vi "REQ-REP.vi"() -> ()   [LabVIEW 2018]
uses:
  RxTx/CM_RxTx.lvclass
  socket REQ/socket REQ.lvclass
  C:/Users/Denis/Desktop/communication-manager/communication-manager/Socket/Socket.lvclass
  socket REP/socket REP.lvclass
  Socket/Socket.lvclass
  <vilib>/addons/zeromq/zmq_context.lvclass
panel:
  in  "socket REP.lvclass":refnum<class "socket REP.lvclass">
  in  "socket REQ.lvclass":refnum<class "socket REQ.lvclass">
  out "error out 3":errorcluster
  in  "Queue RX 2":refnum<class "CM_RxTx.lvclass">
  out "Received message":string
  out "error out 2":errorcluster
  in  "Queue RX":refnum<class "CM_RxTx.lvclass">
  in  "stop":bool
  in  "message":string
  in  "send":bool
  # "REQ endpoint"
  # "REP endpoint"
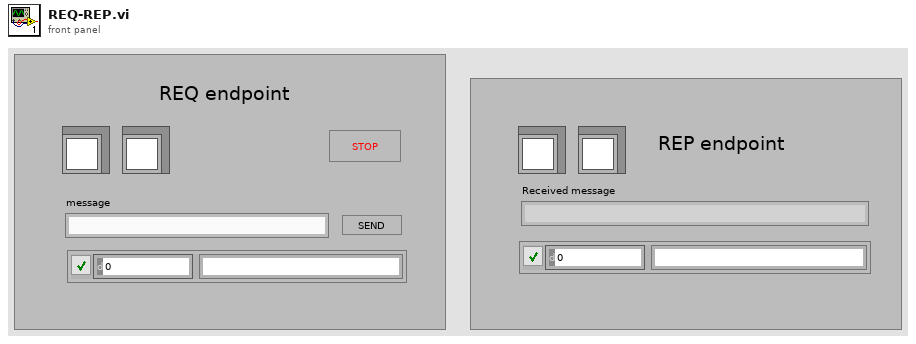
[diagram p1: front panel]
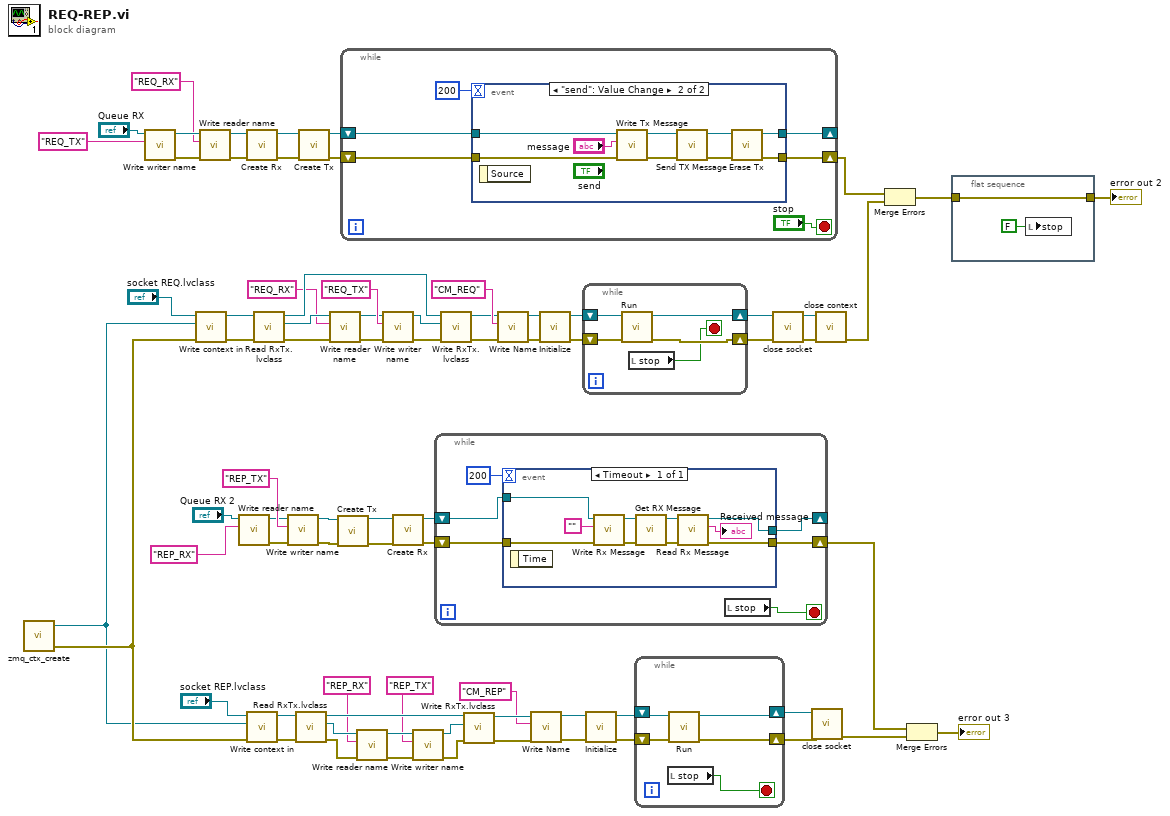
[diagram p0: block diagram]
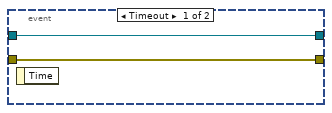
[diagram p2: hidden frame]
diagram:
  n1 = call <vilib>:"zmq_ctx_create.vi"() -> ("error out"=w31:errorcluster, "context out"=w30:refnum<class "zmq_context.lvclass">)  [unwired: 4 in]
  n2 = call-dynamic "Write writer name.vi"("Tx name"="REQ_TX", "RxTx in"="Queue RX") -> ("error out"=w14:errorcluster, "RxTx out"=w13:refnum<class "CM_RxTx.lvclass">)  [unwired: 8 in]
  n3 = call-dynamic "Write context in.vi"("error in (no error)"=w31, "zeromq.lvlib:ZeroMQ Context"=w30, "Socket in"="socket REQ.lvclass") -> ("error out"=w51:errorcluster, "Socket out"=w50:refnum<class "socket REQ.lvclass">)  [unwired: 7 in]
  n4 = call-dynamic "Write reader name.vi"("error in (no error)"=w14, "RX name"="REQ_RX" ("Tx name"), "RxTx in"=w13) -> ("error out"=w16:errorcluster, "RxTx out"=w15:refnum<class "CM_RxTx.lvclass">)  [unwired: 7 in]
  n5 = call-dynamic "Write reader name.vi"("RX name"="REP_RX" ("string"), "RxTx in"="Queue RX 2") -> ("error out"=w7:errorcluster, "RxTx out"=w4:refnum<class "CM_RxTx.lvclass">)  [unwired: 8 in]
  n6 = call "Create Rx.vi"("error in (no error)"=w16, "RxTx in"=w15) -> ("error out"=w18:errorcluster, "RxTx out"=w17:refnum<class "CM_RxTx.lvclass">)  [unwired: 8 in]
  n7 = call-dynamic "Write context in.vi"("error in (no error)"=w31, "zeromq.lvlib:ZeroMQ Context"=w30, "Socket in"="socket REP.lvclass") -> ("error out"=w34:errorcluster, "Socket out"=w35:refnum<class "socket REP.lvclass">)  [unwired: 7 in]
  n8 = call-dynamic "Read RxTx.lvclass.vi"("error in (no error)"=w51, "Socket in"=w50) -> ("error out"=w64:errorcluster, "RxTx.lvclass"=w68:refnum<class "CM_RxTx.lvclass">, "Socket out"=w65:refnum<class "socket REQ.lvclass">)  [unwired: 7 in]
  n9 = call-dynamic "Write writer name.vi"("error in (no error)"=w7, "Tx name"="REP_TX" ("string"), "RxTx in"=w4) -> ("error out"=w6:errorcluster, "RxTx out"=w5:refnum<class "CM_RxTx.lvclass">)  [unwired: 7 in]
  n10 = call-dynamic "Read RxTx.lvclass.vi"("error in (no error)"=w34, "Socket in"=w35) -> ("error out"=w42:errorcluster, "RxTx.lvclass"=w38:refnum<class "CM_RxTx.lvclass">, "Socket out"=w41:refnum<class "socket REP.lvclass">)  [unwired: 7 in]
  n11 = call "Create Tx.vi"("error in (no error)"=w18, "RxTx in"=w17) -> ("error out"=w73:errorcluster, "RxTx out"=w75:refnum<class "CM_RxTx.lvclass">)  [unwired: 8 in]
  n12 = call-dynamic "Write reader name.vi"("error in (no error)"=w64, "RX name"="REQ_RX" ("reader name"), "RxTx in"=w68) -> ("error out"=w63:errorcluster, "RxTx out"=w67:refnum<class "CM_RxTx.lvclass">)  [unwired: 7 in]
  n13 = call "Create Tx.vi"("error in (no error)"=w6, "RxTx in"=w5) -> ("error out"=w8:errorcluster, "RxTx out"=w9:refnum<class "CM_RxTx.lvclass">)  [unwired: 8 in]
  n14 = while {
    shift-right: [w78] -> _
    shift-left: w75 -> [w80]
    shift-right: [w77] -> w49
    shift-left: w73 -> [w79]
    stop <- "stop" stop-if-true
    n15 = event shown="[1] \"send\": Value Change" {
      selector: _ -> [_ _]
      dyn-events: _ -> [_ _]
      timeout: 200 -> [_ _]
      tunnel: [w83 w89] -> w78
      tunnel: [w82 w88] -> w77
      tunnel: w80 -> [w83 w85]
      tunnel: w79 -> [w82 w84]
      event Timeout {
        n16 = event-data() -> ()  [unwired: 1 in, 1 out]
      }
      event "send": Value Change {
        n17 = event-data() -> ()  [unwired: 1 in, 1 out]
        n18 = call "Write Tx Message.vi"("error in (no error)"=w84, "Tx Message"="message", "RxTx in"=w85) -> ("error out"=w86:errorcluster, "RxTx out"=w91:refnum<class "CM_RxTx.lvclass">)  [unwired: 7 in]
        n19 = call "Send TX Message.vi"("error in (no error)"=w86, "RxTx in"=w91) -> ("error out"=w87:errorcluster, "RxTx out"=w90:refnum<class "CM_RxTx.lvclass">)  [unwired: 8 in]
        n20 = call "Erase Tx.vi"("error in (no error)"=w87, "RxTx in"=w90) -> ("error out"=w88:errorcluster, "RxTx out"=w89:refnum<class "CM_RxTx.lvclass">)  [unwired: 8 in]
      }
    }
  }
  n21 = call-dynamic "Write reader name.vi"("error in (no error)"=w42, "RX name"="REP_RX" ("reader name"), "RxTx in"=w38) -> ("error out"=w43:errorcluster, "RxTx out"=w39:refnum<class "CM_RxTx.lvclass">)  [unwired: 7 in]
  n22 = call-dynamic "Write writer name.vi"("error in (no error)"=w63, "Tx name"="REQ_TX" ("writer name"), "RxTx in"=w67) -> ("error out"=w62:errorcluster, "RxTx out"=w66:refnum<class "CM_RxTx.lvclass">)  [unwired: 7 in]
  n23 = call "Create Rx.vi"("error in (no error)"=w8, "RxTx in"=w9) -> ("error out"=w24:errorcluster, "RxTx out"=w25:refnum<class "CM_RxTx.lvclass">)  [unwired: 8 in]
  n24 = call-dynamic "Write writer name.vi"("error in (no error)"=w43, "Tx name"="REP_TX" ("writer name"), "RxTx in"=w39) -> ("error out"=w44:errorcluster, "RxTx out"=w40:refnum<class "CM_RxTx.lvclass">)  [unwired: 7 in]
  n25 = while {
    shift-right: [w96] -> _
    shift-left: w25 -> [w97]
    shift-right: [w94] -> w22
    shift-left: w24 -> [w95]
    stop <- w93 stop-if-true
    n26 = event shown="[0] Timeout" {
      selector: _ -> [_]
      dyn-events: _ -> [_]
      timeout: 200 -> [_]
      tunnel: w97 -> [w105]
      tunnel: [w103] -> w96
      tunnel: w95 -> [w100]
      tunnel: [w99] -> w94
      event Timeout {
        n27 = event-data() -> ()  [unwired: 1 in, 1 out]
        n28 = call "Write Rx Message.vi"("error in (no error)"=w100, "Rx Message"="", "RxTx in"=w105) -> ("error out"=w102:errorcluster, "RxTx out"=w104:refnum<class "CM_RxTx.lvclass">)  [unwired: 7 in]
        n29 = call "Get RX Message.vi"("error in (no error)"=w102, "RxTx in"=w104) -> ("error out"=w106:errorcluster, "RxTx out"=w108:refnum<class "CM_RxTx.lvclass">)  [unwired: 7 in, 1 out]
        n30 = call "Read Rx Message.vi"("error in (no error)"=w106, "RxTx in"=w108) -> ("error out"=w99:errorcluster, "Rx Message"=→"Received message":string, "RxTx out"=w103:refnum<class "CM_RxTx.lvclass">)  [unwired: 7 in]
      }
    }
    n31 = local read "stop"() -> (w93:bool)
  }
  n32 = call-dynamic "Write RxTx.lvclass.vi"("error in (no error)"=w62, "RxTx.lvclass"=w66, "Socket in"=w65) -> ("error out"=w52:errorcluster, "Socket out"=w53:refnum<class "socket REQ.lvclass">)  [unwired: 7 in]
  n33 = call-dynamic "Write RxTx.lvclass.vi"("error in (no error)"=w44, "RxTx.lvclass"=w40, "Socket in"=w41) -> ("error out"=w47:errorcluster, "Socket out"=w46:refnum<class "socket REP.lvclass">)  [unwired: 7 in]
  n34 = call-dynamic "Write Name.vi"("error in (no error)"=w52, "Name"="CM_REQ", "Socket in"=w53) -> ("error out"=w60:errorcluster, "Socket out"=w61:refnum<class "socket REQ.lvclass">)  [unwired: 7 in]
  n35 = call-dynamic "Write Name.vi"("error in (no error)"=w47, "Name"="CM_REP", "Socket in"=w46) -> ("error out"=w32:errorcluster, "Socket out"=w33:refnum<class "socket REP.lvclass">)  [unwired: 7 in]
  n36 = call-dynamic "Initialize.vi"("error in (no error)"=w60, "socket REQ in"=w61) -> ("error out"=w57:errorcluster, "socket REQ out"=w59:refnum<class "socket REQ.lvclass">)  [unwired: 8 in]
  n37 = while {
    shift-right: [w111] -> w58
    shift-left: w59 -> [w113]
    shift-right: [w110] -> w56
    shift-left: w57 -> [w112]
    stop <- w109 stop-if-true
    n38 = call-dynamic "Run.vi"("error in (no error)"=w112, "socket REQ in"=w113) -> ("error out"=w110:errorcluster, "socket REQ out"=w111:refnum<class "socket REQ.lvclass">)  [unwired: 8 in]
    n39 = local read "stop"() -> (w109:bool)
  }
  n40 = call-dynamic "Initialize.vi"("error in (no error)"=w32, "socket REP in"=w33) -> ("error out"=w28:errorcluster, "socket REP out"=w29:refnum<class "socket REP.lvclass">)  [unwired: 8 in]
  n41 = while {
    shift-right: [w116] -> w26
    shift-left: w29 -> [w118]
    shift-right: [w115] -> w27
    shift-left: w28 -> [w117]
    stop <- w114 stop-if-true
    n42 = local read "stop"() -> (w114:bool)
    n43 = call-dynamic "Run.vi"("error in (no error)"=w117, "socket REP in"=w118) -> ("error out"=w115:errorcluster, "socket REP out"=w116:refnum<class "socket REP.lvclass">)  [unwired: 8 in]
  }
  n44 = call "close socket.vi"("error in (no error)"=w56, "Socket in"=w58) -> ("error out"=w71:errorcluster, "Socket out"=w70:refnum<class "socket REQ.lvclass">)  [unwired: 8 in]
  n45 = call "close socket.vi"("error in (no error)"=w27, "Socket in"=w26) -> ("error out"=w21:errorcluster)  [unwired: 8 in, 1 out]
  n46 = call-dynamic "close context.vi"("error in (no error)"=w71, "Socket in"=w70) -> ("error out"=w48:errorcluster)  [unwired: 8 in, 1 out]
  n47 = Merge Errors(w49, w48) -> (w2:errorcluster)
  n48 = Merge Errors(w22, w21) -> (→"error out 3":errorcluster)
  n49 = flat-sequence {
    tunnel: w2 -> [w120]
    tunnel: [w120] -> w1
    frame #0 {
      n50 = local write "stop"(FALSE ("stop")) -> ()
    }
  }
  "error out 2" <- w1
